vi "1D I32 Array_DeleteCellsWithSpecifiedValue.vi"(1 "CellValueToBeDeleted":i32, 2 "1D I32 Array.IN":i32[](array[numeric])=[0, 0]) -> (6 "1D I32 Array.OUT":i32[](array[numeric]))   [LabVIEW 2024]
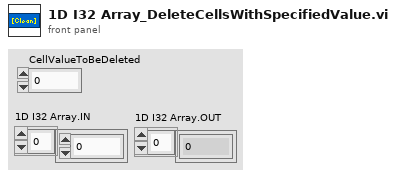
[diagram p1: front panel]
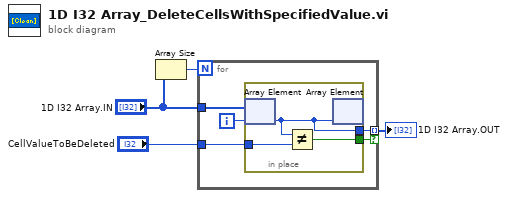
[diagram p0: block diagram]
diagram:
  n1 = Array Size(array="1D I32 Array.IN") -> (size(s)=w4:i32)
  n2 = for {
    N: w4 -> [_]
    tunnel: "1D I32 Array.IN" -> [w9]
    tunnel: [w7] -> w2 mode=indexing if=w5
    tunnel: "CellValueToBeDeleted" -> [w6]
    i -> [w8]
    n3 = in-place {
      in-place-border: [w11] -> w7
      in-place-border: w6 -> [w12]
      in-place-border: [w10] -> w5
      n4 = in-place-array #1(w9, w8) -> (w11:i32)
      n5 = Not Equal?(x=w11, y=w12) -> (x != y?=w10:bool)
      n6 = in-place-array #1(w11) -> ()  [unwired: 2 out]
    }
  }
  "1D I32 Array.OUT" <- w2
